vi "extract active channels.vi"(7 "RT Queues":T1, 9 "Data":T2={"Parameters"={"FPGA Ref"=refnum, "data stream"={"data writer name"="error writer", "NS write buffer size"=16, "NS Buffer length"=0}, "FIFO Depth"=0, "Channel controls"={"FIFO channel count"=0, "active indices"=[], "active channels"=0, "channelScaling"=[], "scanivalveCount"=0, "channels"=[]}, "safetyChannels"={"oilP"=0, "airP"=0, "water"=0, "channelLimits"=[]}, "speedChannel"=0, "maxSpeedLimit"=0.0, "Torque"={"fixedOffset"=0.0, "filter"=FALSE, "fallingEdge"=FALSE, "swapEncoders"=FALSE}}, "Variables"={"Intermediary buffer"=[], "buffer position"=0, "write loop counter"=0, "NS write trigger"=0, "NS Connection status"=FALSE, "waiting for NS"=FALSE, "labAmbient"={"pressure"=0.0, "temperature"=0.0}, "scanivalvePorts"=[], "scanivalvePressures"=[], "data stream"="", "activeChannelLimitIndex"=[], "runningSpeedLimit"=0.0, "speedChannelIndex"=0, "Interlocks"={"gearboxOil"=FALSE, "bearingOil"=FALSE, "gearboxAir"=FALSE}, "interlockChannels"={"gearboxOil"=0, "bearingOil"=0, "air"=0}, "limitStates"=[]}}, 11 "Data in":variant) -> (1 "Data out":T2={"Parameters"={"FPGA Ref"=refnum, "data stream"={"data writer name"="error writer", "NS write buffer size"=16, "NS Buffer length"=0}, "FIFO Depth"=0, "Channel controls"={"FIFO channel count"=0, "active indices"=[], "active channels"=0, "channelScaling"=[], "scanivalveCount"=0, "channels"=[]}, "safetyChannels"={"oilP"=0, "airP"=0, "water"=0, "channelLimits"=[]}, "speedChannel"=0, "maxSpeedLimit"=0.0, "Torque"={"fixedOffset"=0.0, "filter"=FALSE, "fallingEdge"=FALSE, "swapEncoders"=FALSE}}, "Variables"={"Intermediary buffer"=[], "buffer position"=0, "write loop counter"=0, "NS write trigger"=0, "NS Connection status"=FALSE, "waiting for NS"=FALSE, "labAmbient"={"pressure"=0.0, "temperature"=0.0}, "scanivalvePorts"=[], "scanivalvePressures"=[], "data stream"="", "activeChannelLimitIndex"=[], "runningSpeedLimit"=0.0, "speedChannelIndex"=0, "Interlocks"={"gearboxOil"=FALSE, "bearingOil"=FALSE, "gearboxAir"=FALSE}, "interlockChannels"={"gearboxOil"=0, "bearingOil"=0, "air"=0}, "limitStates"=[]}}, 3 "Active channels":dbl[][](array[numeric]))   [LabVIEW 2018]
uses:
  Type Defs/Data processing loop data.ctl
  Type Defs/FPGA reference.ctl
  PC/type defs/channelControl.ctl
  Type Defs/channelScalingTypes.ctl
  Type Defs/scalingMethods.ctl
  ICL-LabVIEW_General/data channels/parent class/Data Channel.lvclass
  PC/type defs/channelLimitControl.ctl
  PC/type defs/limitActions.ctl
  Type Defs/Queues cluster.ctl
  ICL-LabVIEW_General/Message Scheduler/message scheduler.lvclass
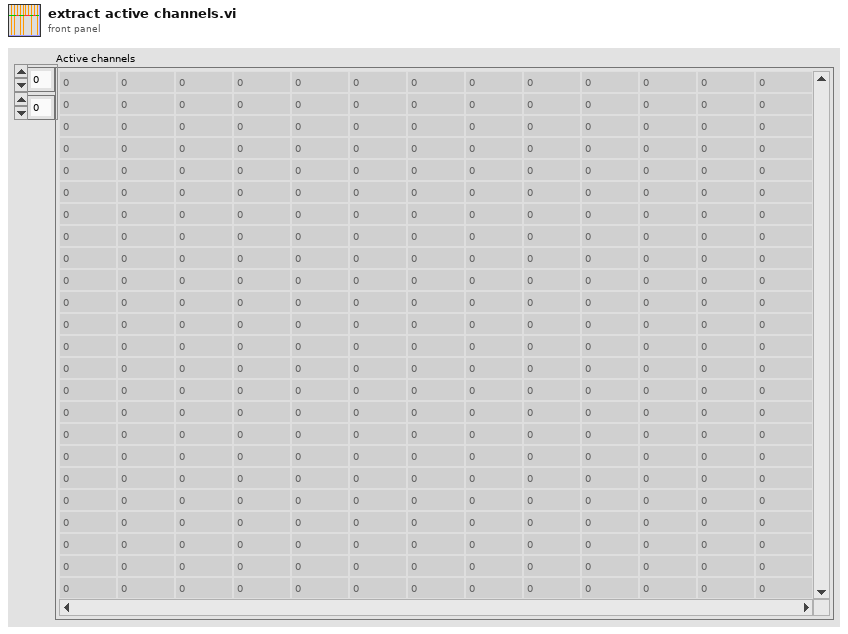
[diagram p1: front panel]
types:
  T1 = typedef "Queues cluster.ctl" = cluster{"RT Message":refnum<queue>, "RT Comms":refnum<queue>, "RT Data":refnum<queue>, "RT FIFO":refnum<queue>, "message scheduler":refnum<class "message scheduler.lvclass">}
  T2 = typedef "Data processing loop data.ctl" = cluster{"Parameters":cluster{"FPGA Ref":T3, "data stream":cluster{"data writer name":string, "NS write buffer size":i32, "NS Buffer length":u32}, "FIFO Depth":u32, "Channel controls":cluster{"FIFO channel count":i32, "active indices":i16[], "active channels":i32, "channelScaling":T4[], "scanivalveCount":i32, "channels":refnum<class "Data Channel.lvclass">[]}, "safetyChannels":cluster{"oilP":u16, "airP":u16, "water":u16, "channelLimits":T7[]}, "speedChannel":i32, "maxSpeedLimit":dbl, "Torque":cluster{"fixedOffset":dbl, "filter":bool, "fallingEdge":bool, "swapEncoders":bool}}, "Variables":cluster{"Intermediary buffer":dbl[][], "buffer position":u32, "write loop counter":u16, "NS write trigger":u32, "NS Connection status":bool, "waiting for NS":bool, "labAmbient":cluster{"pressure":dbl, "temperature":dbl}, "scanivalvePorts":u16[], "scanivalvePressures":dbl[], "data stream":refnum<k21>, "activeChannelLimitIndex":u16[], "runningSpeedLimit":dbl, "speedChannelIndex":i32, "Interlocks":cluster{"gearboxOil":bool, "bearingOil":bool, "gearboxAir":bool}, "interlockChannels":cluster{"gearboxOil":i32, "bearingOil":i32, "air":i32}, "limitStates":cluster{"warn":bool, "alarm":bool}[]}}
  T3 = typedef "FPGA reference.ctl" = refnum<k20>
  T4 = typedef "channelControl.ctl" = cluster{"index":u16, "active":bool, "channelType":T5, "module":u16, "terminal":u16, "channelName":string, "scalingMethod":T6, "scalingParameters":dbl[], "scaledUnits":string, "tempOffset":dbl}
  T5 = typedef "channelScalingTypes.ctl" = enum16{"calculation", "measurement", "scanivalve", "output", "digital"}
  T6 = typedef "scalingMethods.ctl" = enum16{"none", "linear", "thermocouple", "polynomial", "encoder", "RTD"}
  T7 = typedef "channelLimitControl.ctl" = cluster{"channelID":u16, "Enabled":bool, "warnValue":dbl, "limitValue":dbl, "Invert":bool, "limitAction":T8}
  T8 = typedef "limitActions.ctl" = enum16{"stop", "shutdown", "ignore"}
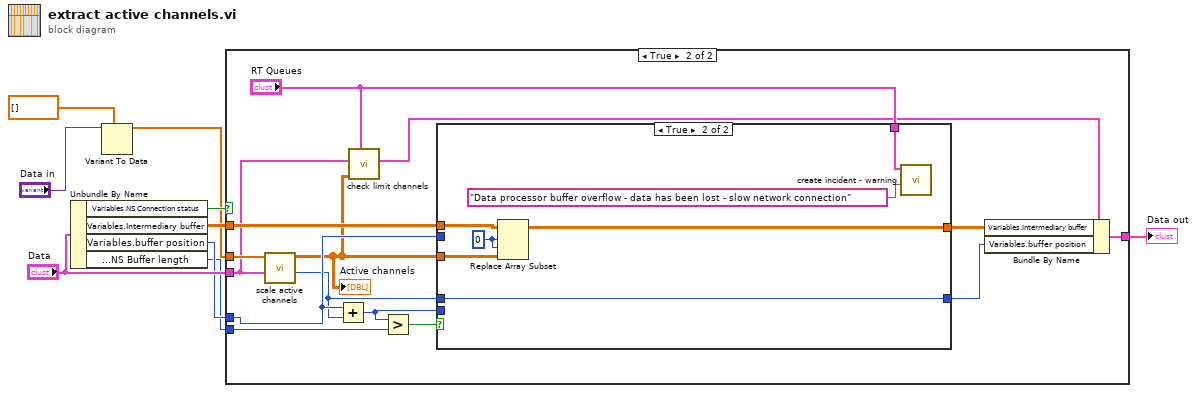
[diagram p0: block diagram]
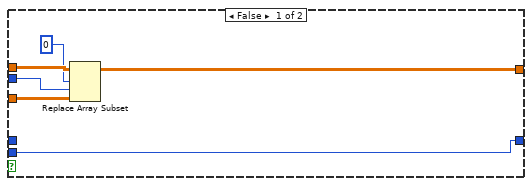
[diagram p3: hidden frame]
diagram:
  n1 = Unbundle By Name("Data") -> ("Variables.NS Connection status"=w3:bool, "Variables.Intermediary buffer"=w6:dbl[][], "Variables.buffer position"=w4:u32, "Parameters.data stream.NS Buffer length"=w2:u32)
  n2 = Variant To Data(type=sgl[] [] ("Data"), Variant="Data in") -> (data=w1:sgl[])  [unwired: 1 in, 1 out]
  n3 = case shown="True" w3 {
    tunnel: "Data" -> [w10 w14]
    tunnel: w6 -> [_ w24]
    tunnel: [w10 w23] -> w5
    tunnel: w4 -> [_ w19]
    tunnel: w2 -> [_ w20]
    tunnel: w1 -> [_ w18]
    frame False {
      # "Don't put anything in the buffer if the network stream is not connected"
    }
    frame True {
      n4 = call "scale active channels.vi"("input cluster"=w14, "raw data"=w18) -> ("data length"=w15:i32, "Active channels"=w13:dbl[][])  [unwired: 8 in]
      "Active channels" <- w13
      n5 = Add(x=w19, y=w15) -> (x+y=w16:u32)
      n6 = call "check limit channels.vi"("RT Queues in"="RT Queues", "Active channels"=w13, "Data"=w14) -> ("Data out"=w11:T2)  [unwired: 8 in]
      n7 = Greater?(x=w16, y=w20) -> (0:w17:bool)
      n8 = case shown="True" w17 {
        tunnel: w24 -> [w30 w37]
        tunnel: w13 -> [w29 w36]
        tunnel: [w28 w35] -> w22
        tunnel: w19 -> [w25 _]
        tunnel: w15 -> [_ w33]
        tunnel: w16 -> [w27 _]
        tunnel: [w27 w33] -> w21
        tunnel: "RT Queues" -> [_ w31]
        frame False {
          n9 = Replace Array Subset(array=w30, new element=w29, index (row)=0 ("disabled index (col)"), index (col)=w25) -> (w28:dbl[][])
        }
        frame True {
          w34 = 0 ("disabled index (col)")
          n10 = Replace Array Subset(array=w37, new element=w36, index (row)=w34, index (col)=w34) -> (w35:dbl[][])
          n11 = call "create incident - warning.vi"("warning description"="Data processor buffer overflow - data has been lost - slow network connection" ("Description"), "RT Queues"=w31) -> ()  [unwired: 9 in, 1 out]
        }
      }
      n12 = Bundle By Name(cluster=w11, "Variables.Intermediary buffer"=w22, "Variables.buffer position"=w21) -> (w23:T2)
    }
  }
  "Data out" <- w5
